vi "SetPointSparkMax.vi"(6 "Time To Run (S)":dbl, 8 "Deadband":dbl, 9 "Timeout In":dbl, 10 "MotorControlDeviceRef":T1, 11 "Setpoint":dbl) -> (3 "Is Finished?":bool)   [LabVIEW 2020]
uses:
  <vilib>/Rock Robotics/WPI/MotorControl/WPI_MotorControlDeviceRef.ctl
  <vilib>/Rock Robotics/WPI/MotorControl/WPI_MotorControlType.ctl
  <vilib>/Rock Robotics/SystemInterfaces/DIO/FPGA_DIOPWMChannel.ctl
  <vilib>/Rock Robotics/WPI/PWM/WPI_PWMDeadband.ctl
  <vilib>/Rock Robotics/SystemInterfaces/DIO/FPGA_DIOChannel.ctl
  <vilib>/Rock Robotics/WPI/ThirdParty/REV Robotics/REVLib/Typedef/Spark MAX Control Type.ctl
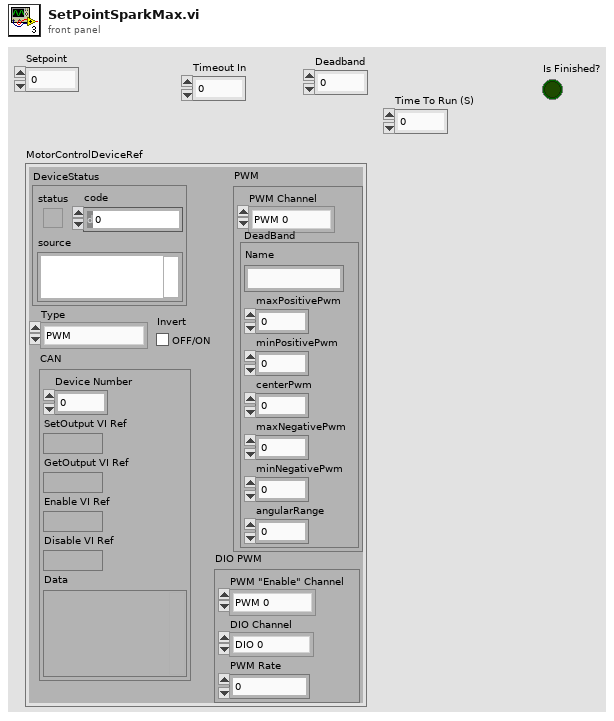
[diagram p1: front panel]
types:
  T1 = typedef "WPI_MotorControlDeviceRef.ctl" = cluster{"DeviceStatus":errorcluster, "Type":T2, "PWM":cluster{"PWM Channel":T3, "DeadBand":T4}, "CAN":cluster{"Device Number":u8, "SetOutput VI Ref":variant, "GetOutput VI Ref":variant, "Enable VI Ref":variant, "Disable VI Ref":variant, "Data":variant}, "Invert":bool, "DIO PWM":cluster{"PWM \"Enable\" Channel":T3, "DIOChannel":T5, "PWM Rate":dbl}}
  T2 = typedef "WPI_MotorControlType.ctl" = enum16{"PWM", "CAN", "DIO PWM"}
  T3 = typedef "FPGA_DIOPWMChannel.ctl" = enum8{"PWM 0", "PWM 1", "PWM 2", "PWM 3", "PWM 4", "PWM 5", "PWM 6", "PWM 7", "PWM 8", "PWM 9", "PWM MXP 0", "PWM MXP 1", "PWM MXP 2", "PWM MXP 3", "PWM MXP 4", "PWM MXP 5", "PWM MXP 6", "PWM MXP 7", "PWM MXP 8", "PWM MXP 9", "Invalid"}
  T4 = typedef "WPI_PWMDeadband.ctl" = cluster{"Name":string, "maxPositivePwm":i32, "minPositivePwm":i32, "centerPwm":i32, "maxNegativePwm":i32, "minNegativePwm":i32, "angularRange":u16}
  T5 = typedef "FPGA_DIOChannel.ctl" = enum8{"DIO 0", "DIO 1", "DIO 2", "DIO 3", "DIO 4", "DIO 5", "DIO 6", "DIO 7", "DIO 8", "DIO 9", "DIO MXP 0", "DIO MXP 1", "DIO MXP 2", "DIO MXP 3", "DIO MXP 4", "DIO MXP 5", "DIO MXP 6", "DIO MXP 7", "DIO MXP 8", "DIO MXP 9", "DIO MXP 10", "DIO MXP 11", "DIO MXP 12", "DIO MXP 13", "DIO MXP 14", "DIO MXP 15", "SPI Port CS1", "SPI Port CS2", "SPI Port CS3", "SPI Port MISO", "SPI Port MOSI", "Invalid"}
  T6 = typedef "Spark MAX Control Type.ctl" = enum16{"Percent VBus", "Voltage", "Velocity", "Position", "Smart Motion", "Current", "Smart Velocity"}
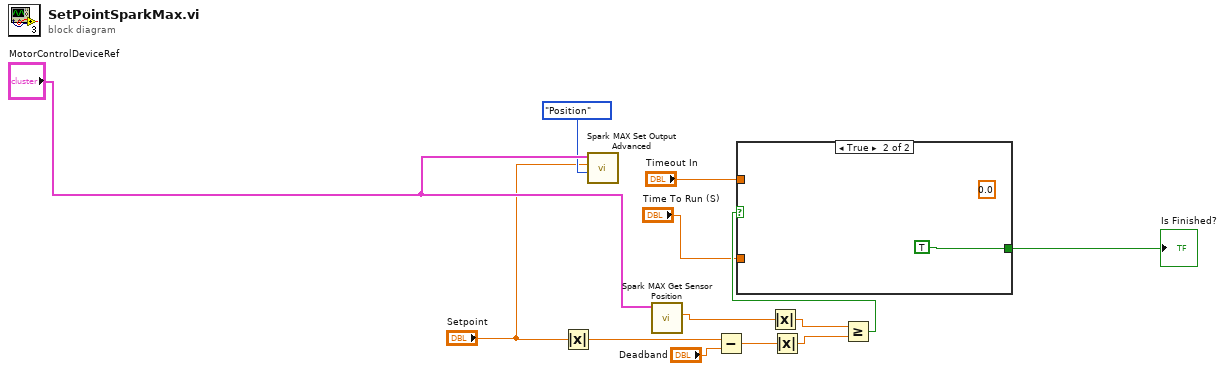
[diagram p0: block diagram]
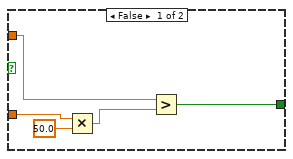
[diagram p2: hidden frame]
diagram:
  n1 = Absolute Value(x="Setpoint") -> (abs(x)=w1:dbl)
  n2 = call <vilib>:"Spark MAX Set Output Advanced.vi"("Control Mode"=Spark_MAX_Control_Type."Position", "Setpoint"="Setpoint", "MotorControlDevRef"="MotorControlDeviceRef") -> ()  [unwired: 7 in, 2 out]
  n3 = call <vilib>:"Spark MAX Get Sensor Position.vi"("MotorControlDevRef in"="MotorControlDeviceRef") -> ("Sensor Position"=w9:dbl)  [unwired: 7 in, 3 out]
  n4 = Subtract(x=w1, y="Deadband") -> (x-y=w10:dbl)
  n5 = Absolute Value(x=w9) -> (abs(x)=w8:dbl)
  n6 = Absolute Value(x=w10) -> (abs(x)=w7:dbl)
  n7 = Greater Or Equal?(x=w8, y=w7) -> (x >= y?=w6:bool)
  n8 = case shown="True" w6 {
    tunnel: [w18 TRUE ("Is Finished?")] -> w12
    tunnel: "Timeout In" -> [w17 _]
    tunnel: "Time To Run (S)" -> [w15 _]
    frame False {
      n9 = Multiply(x=w15, y=50.0) -> (x*y=w14:dbl)
      n10 = Greater?(x=w17, y=w14) -> (0:w18:bool)
    }
    frame True {
      (unwired) 0.0
    }
  }
  "Is Finished?" <- w12
